vi "Elevator Control Loop.vi"() -> ()   [LabVIEW 2014, in "Elevator System.lvlib"]
uses:
  Elevator System.lvlib
  <vilib>/addons/control/pid/NI_PID_pid.lvlib
  <vilib>/addons/control/pid/pid.llb/PID (DBL).vi
  <vilib>/Rock Robotics/WPI/PWM/WPI_PWMTransform_ConPane.ctl
  <vilib>/Rock Robotics/WPI/CAN/TalonSRX/WPI_CANTalonSRX_APIControlMode.ctl
  <vilib>/Rock Robotics/WPI/CAN/Jaguar/SubVIs/WPI_CANJaguar_ControlMode.ctl
  <vilib>/Rock Robotics/WPI/PWM/WPI_PWMDeadband.ctl
  <vilib>/Rock Robotics/SystemInterfaces/DIO/FPGA_DIOPWMChannel.ctl
  <vilib>/Rock Robotics/SystemInterfaces/Typedef/FPGA_TypedefDigitalModule.ctl
  <vilib>/Rock Robotics/WPI/MotorControl/WPI_MotorControlType.ctl
  <vilib>/Rock Robotics/WPI/MotorControl/WPI_MotorControlDeviceRef.ctl
  SimulatorVIs/Simulation Input Global.vi
  Typedef/FGVAction.ctl
panel:
  out "Plant Input":dbl(graph)
  in  "output range":cluster{"output high":dbl, "output low":dbl}={"output high"=100.0, "output low"=-1.0} {"output low" format="%.2f"; "output high" format="%.2f"}
  in  "PID gains":T1={"proportional gain (Kc)"=11.9, "integral time (Ti, min)"=0.004, "derivative time (Td, min)"=0.0} {"derivative time (Td, min)" format="%.3f"; "integral time (Ti, min)" format="%.3f"; "proportional gain (Kc)" format="%.3f"}
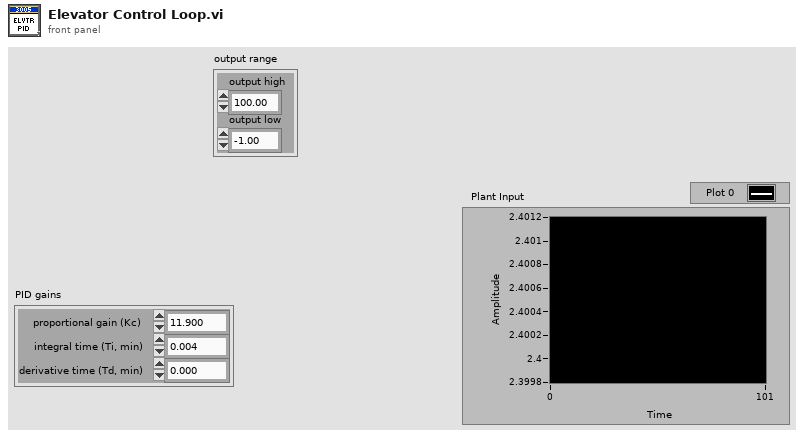
[diagram p1: front panel]
types:
  T1 = cluster{"proportional gain (Kc)":dbl, "integral time (Ti, min)":dbl, "derivative time (Td, min)":dbl}
  T2 = typedef "WPI_MotorControlDeviceRef.ctl" = cluster{"DeviceStatus":errorcluster, "Type":T3, "PWM":cluster{"Controller":T4, "PWM Channel":T5, "DeadBand":T6}, "CAN":cluster{"Device Number":u8, "Control Mode":T7, "Semaphore":T8, "Max Vout":dbl, "TalonSRX Control Mode":T9}, "Invert":bool, "TransformRef":T10, "InvTransformRef":T10}
  T3 = typedef "WPI_MotorControlType.ctl" = enum16{"PWM", "CAN", "CANTalonSRX"}
  T4 = typedef "FPGA_TypedefDigitalModule.ctl" = enum16{"Controller 1"}
  T5 = typedef "FPGA_DIOPWMChannel.ctl" = enum8{"PWM 0", "PWM 1", "PWM 2", "PWM 3", "PWM 4", "PWM 5", "PWM 6", "PWM 7", "PWM 8", "PWM 9", "PWM MXP 0", "PWM MXP 1", "PWM MXP 2", "PWM MXP 3", "PWM MXP 4", "PWM MXP 5", "PWM MXP 6", "PWM MXP 7", "PWM MXP 8", "PWM MXP 9", "Invalid"}
  T6 = typedef "WPI_PWMDeadband.ctl" = cluster{"Name":string, "maxPositivePwm":i32, "minPositivePwm":i32, "centerPwm":i32, "maxNegativePwm":i32, "minNegativePwm":i32, "angularRange":u16}
  T7 = typedef "WPI_CANJaguar_ControlMode.ctl" = enum8{"Percent VBus", "Current", "Speed", "Position", "Voltage"}
  T8 = typedef "Semaphore RefNum" = refnum<k1>
  T9 = typedef "WPI_CANTalonSRX_APIControlMode.ctl" = enum8{"Percent VBus", "Speed", "Position", "Slave", "Unchanged / Invalid"}
  T10 = typedef "WPI_PWMTransform_ConPane.ctl" = refnum<vi>
  T11 = cluster{"Setpoint":dbl, "notifier out":refnum<notifier>, "Output":dbl, "DriveMotor":T2}
  T12 = typedef "Elevator System.lvlib/FGVAction.ctl" = enum16{"get", "set"}
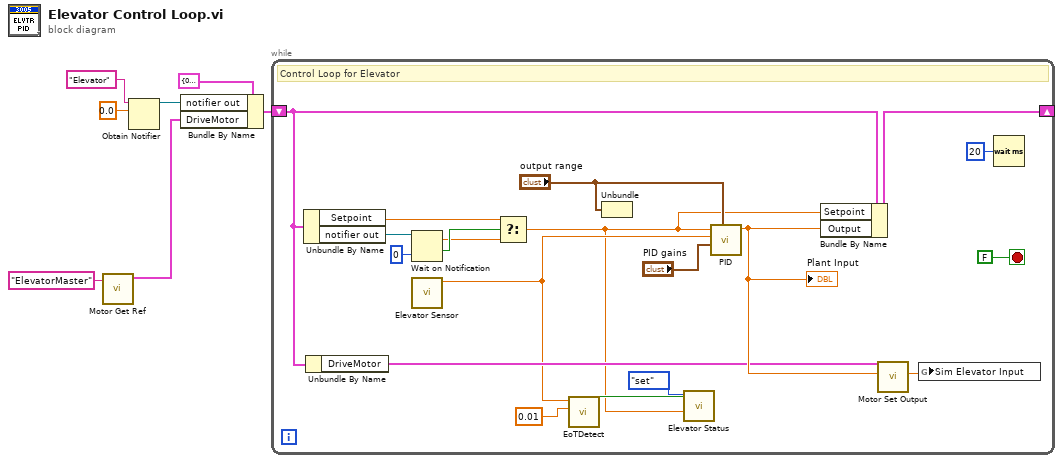
[diagram p0: block diagram]
diagram:
  n1 = call "Motor Get Ref.vi"("refnum name"="ElevatorMaster") -> ("MotorControlDevRef"=w2:T2)  [unwired: 10 in]
  n2 = Obtain Notifier(name (unnamed)="Elevator", notification data type=0.0 ("Setpoint")) -> (notifier out=w5:refnum<notifier>)  [unwired: 2 in, 2 out]
  n3 = Bundle By Name(cluster=T11 {"Setpoint"=0.0, "notifier out"=refnum, "Output"=0.0, "DriveMotor"={"DeviceStatus"={"status"=FALSE, "code"=0, "source"=""}, "Type"=enum."PWM", "PWM"={"Controller"=enum."Controller 1", "PWM Channel"=enum."Invalid", "DeadBand"={"Name"="", "maxPositivePwm"=0, "minPositivePwm"=0, "centerPwm"=0, "maxNegativePwm"=0, "minNegativePwm"=0, "angularRange"=0}}, "CAN"={"Device Number"=0, "Control Mode"=enum."Percent VBus", "Semaphore"=refnum, "Max Vout"=12.0, "TalonSRX Control Mode"=enum."Percent VBus"}, "Invert"=FALSE, "TransformRef"=refnum, "InvTransformRef"=refnum}}, "notifier out"=w5, "DriveMotor"=w2) -> (w6:T11)
  n4 = while {
    shift-right: [w20] -> _
    shift-left: w6 -> [w19]
    stop <- FALSE stop-if-true
    # "Control Loop for Elevator"
    n5 = Unbundle By Name(w19) -> ("Setpoint"=w23:dbl, "notifier out"=w25:refnum<notifier>)
    n6 = Unbundle By Name(w19) -> ("DriveMotor"=w14:T2)
    n7 = Wait on Notification(notifier=w25, timeout in ms (-1)=0) -> (notification=w15:dbl, timed out?=w24:bool)  [unwired: 2 in, 2 out]
    n8 = call "Elevator Sensor.vi"() -> ("Value"=w11:dbl)  [unwired: 10 in, 1 out]
    n9 = Select(t=w23, s=w24, f=w15) -> (s? t:f=w8:dbl)
    n10 = call "EoTDetect.vi"("Tolerance"=0.01, "Sensor"=w11) -> ("EoT? (F)"=w9:bool)  [unwired: 9 in]
    n11 = Unbundle("output range") -> ()  [unwired: 2 out]
    n12 = call "Elevator Status.vi"(9:w8, "Input"=w9, "Moving? (F)"=FGVAction."set" ("Action")) -> ()  [unwired: 6 in, 3 out]
    n13 = call-poly <vilib>:"PID.vi"("output range"="output range", "PID gains"="PID gains", "process variable"=w11, "setpoint"=w8) -> ("output"=w18:dbl)  [unwired: 6 in, 1 out]
    "Plant Input" <- w18
    n14 = Bundle By Name(cluster=w19, "Setpoint"=w8, "Output"=w18) -> (w20:T11)
    n15 = call "Motor Set Output.vi"("output"=w18, "DriveMotor"=w14) -> ("Motor Output"=w13:dbl)  [unwired: 9 in]
    n16 = global write "Simulation Input Global.vi" "Sim Elevator Input"(w13) -> ()
    n17 = Wait (ms)(milliseconds to wait=u32 20) -> ()  [unwired: 1 out]
  }
